vi "Sort Items.vi"(8 "错误输入":errorcluster, 11 "Listbox Ref":refnum<vi>) -> (0 "错误输出":errorcluster, 3 "Dup Listbox Ref":refnum<vi>)   [LabVIEW 2012, in "Listbox Tool.lvlib"]
uses:
  Listbox Tool.lvlib
  Custom Type/Read and Write Mode.ctl
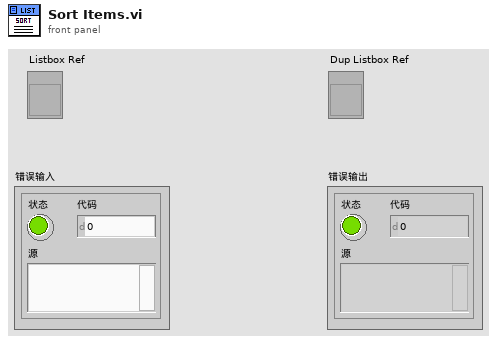
[diagram p1: front panel]
types:
  T1 = typedef "Listbox Tool.lvlib/Read and Write Mode.ctl" = enum16{"Read", "Write"}
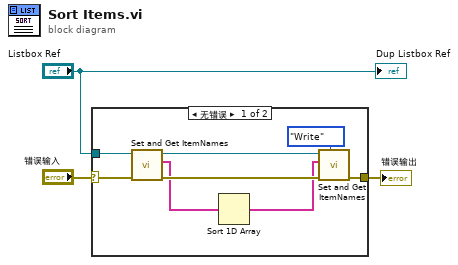
[diagram p0: block diagram]
diagram:
  n1 = case shown="无错误" "错误输入" {
    selector: "错误输入" -> [w11 w12]
    tunnel: "Listbox Ref" -> [w10 _]
    tunnel: [w6 w12] -> w1
    frame No Error {
      n2 = call "Set and Get ItemNames.vi"("错误输入"=w11, "Listbox Ref"=w10) -> ("错误输出"=w9:errorcluster, "ItemNames Out"=w5:string[], "Dup Listbox Ref"=w8:refnum<vi>)  [unwired: 7 in]
      n3 = Sort 1D Array(array=w5) -> (sorted array=w4:string[])
      n4 = call "Set and Get ItemNames.vi"("Mode"=Read_and_Write_Mode."Write", "错误输入"=w9, "ItemNames In"=w4, "Listbox Ref"=w8) -> ("错误输出"=w6:errorcluster)  [unwired: 5 in, 2 out]
    }
    frame Error {
    }
  }
  "错误输出" <- w1
  "Dup Listbox Ref" <- "Listbox Ref"
